vi "Find Car Control VI.vi"(11 "Project":refnum<vi>) -> (0 "error out":errorcluster, 3 "Car Control VI Path":path)   [LabVIEW 2020]
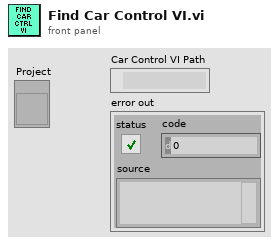
[diagram p1: front panel]
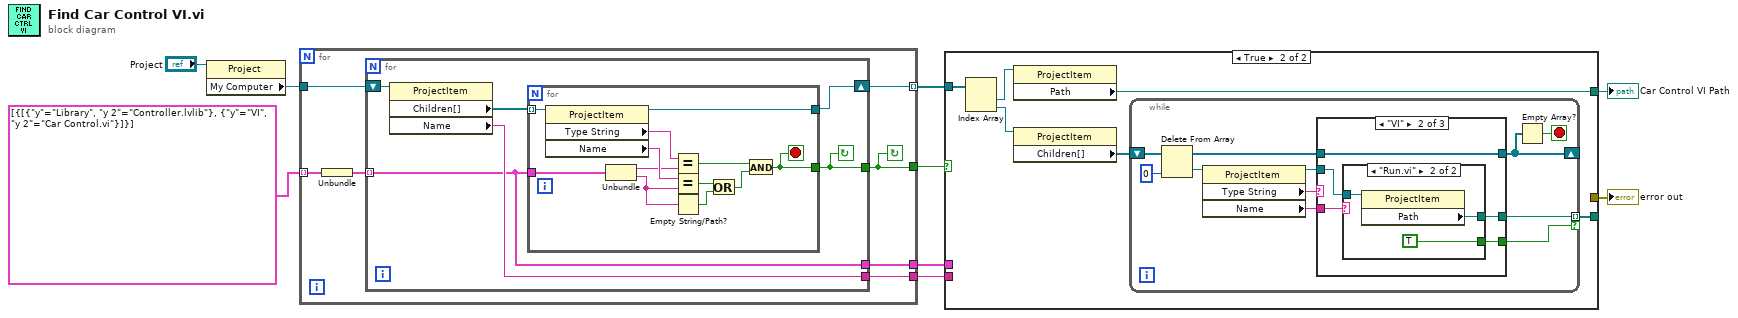
[diagram p0: block diagram]
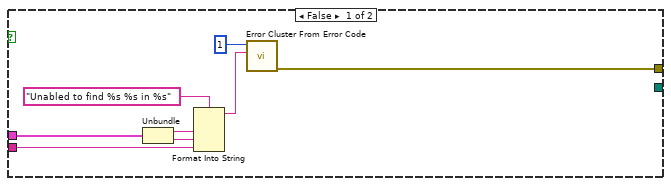
[diagram p2: hidden frame]
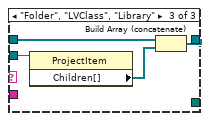
[diagram p5: hidden frame]
diagram:
  n1 = property class="Project"(reference="Project") -> ("My Computer"=w9:refnum<vi>)  [unwired: 1 in, 2 out]
  n2 = for {
    tunnel: w9 -> [w16]
    tunnel: cluster{cluster{"y":string, "y 2":string}[]}[] [{[{"y"="Library", "y 2"="Controller.lvlib"}, {"y"="VI", "y 2"="Car Control.vi"}]}] -> [w15] mode=indexing
    tunnel: [w13] -> w6 mode=indexing
    tunnel: [w12] -> w5
    tunnel: [w11] -> w3
    tunnel: [w10] -> w4
    stop <- w12 continue-if-true
    n3 = Unbundle(w15) -> (w14:cluster{"y":string, "y 2":string}[])
    n4 = for {
      shift-right: [w20] -> w13
      shift-left: w16 -> [w22]
      tunnel: w14 -> [w17] mode=indexing
      tunnel: [w19] -> w12
      tunnel: [w18] -> w11
      tunnel: [w17] -> w10
      stop <- w19 continue-if-true
      n5 = property class="ProjectItem"(reference=w22) -> ("Children[]"=w21:refnum<vi>[], "Name"=w18:string)  [unwired: 1 in, 2 out]
      n6 = for {
        tunnel: w21 -> [w34] mode=indexing
        tunnel: [w32] -> w20
        tunnel: w17 -> [w28]
        tunnel: [w26] -> w19
        stop <- w26 stop-if-true
        n7 = property class="ProjectItem"(reference=w34) -> (reference out=w32:refnum<vi>, "Type String"=w33:string, "Name"=w31:string)  [unwired: 1 in, 1 out]
        n8 = Unbundle(w28) -> ("y"=w27:string, "y 2"=w25:string)
        n9 = Equal?(x=w33, y=w27) -> (x = y?=w30:bool)
        n10 = Equal?(x=w31, y=w25) -> (x = y?=w29:bool)
        n11 = Empty String/Path?(string/path=w25) -> (empty?=w23:bool)
        n12 = Or(x=w29, y=w23) -> (x .or. y?=w24:bool)
        n13 = And(x=w30, y=w24) -> (x .and. y?=w26:bool)
      }
    }
  }
  n14 = case shown="True" w5 {
    tunnel: w6 -> [_ w48]
    tunnel: w4 -> [w40 _]
    tunnel: w3 -> [w37 _]
    tunnel: [w35 _] -> w1
    tunnel: [_ w46] -> w2
    tunnel: [_ w43] -> _
    frame False {
      n15 = Unbundle(w40) -> ("y"=w39:string, "y 2"=w38:string)
      n16 = Format Into String(format string="Unabled to find %s %s in %s", w39, w38, w37) -> (resulting string=w36:string)  [unwired: 2 in, 1 out]
      n17 = call <vilib>:"Error Cluster From Error Code.vi"("error message (\"\")"=w36, "error code (0)"=1) -> ("error out"=w35:errorcluster)  [unwired: 7 in]
    }
    frame True {
      n18 = Index Array(array=w48) -> (element #1=w47:refnum<vi>, element #2=w45:refnum<vi>)  [unwired: 2 in]
      n19 = property class="ProjectItem"(reference=w47) -> ("Path"=w46:path)  [unwired: 1 in, 2 out]
      n20 = property class="ProjectItem"(reference=w45) -> ("Children[]"=w44:refnum<vi>[])  [unwired: 1 in, 2 out]
      n21 = while {
        shift-right: [w53] -> _
        shift-left: w44 -> [w59]
        tunnel: [w50] -> w43 mode=indexing if=w49
        stop <- w52 stop-if-true
        n22 = Delete From Array(array=w59, index=0) -> (deleted portion=w57:refnum<vi>, array with subset deleted=w55:refnum<vi>[])  [unwired: 1 in]
        n23 = property class="ProjectItem"(reference=w57) -> (reference out=w54:refnum<vi>, "Type String"=w56:string, "Name"=w51:string)  [unwired: 1 in, 1 out]
        n24 = case shown="\"VI\"" w56 {
          tunnel: w55 -> [w60 w64 w71]
          tunnel: [w60 w64 w69] -> w53
          tunnel: w54 -> [_ w63 w72]
          tunnel: w51 -> [_ w65 _]
          tunnel: [_ w62 _] -> w50
          tunnel: [_ w61 _] -> w49
          frame Default {
          }
          frame "VI" {
            n25 = case shown="\"Run.vi\"" w65 {
              tunnel: w63 -> [_ w68]
              tunnel: [_ w67] -> w62
              tunnel: [_ TRUE] -> w61
              frame "False", Default {
              }
              frame "Run.vi" {
                n26 = property class="ProjectItem"(reference=w68) -> ("Path"=w67:path)  [unwired: 1 in, 2 out]
              }
            }
          }
          frame "Folder", "LVClass", "Library" {
            n27 = property class="ProjectItem"(reference=w72) -> ("Children[]"=w70:refnum<vi>[])  [unwired: 1 in, 2 out]
            n28 = Build Array (concatenate)(w71, w70) -> (w69:refnum<vi>[])
          }
        }
        n29 = Empty Array?(array=w53) -> (empty?=w52:bool)
      }
    }
  }
  "Car Control VI Path" <- w2
  "error out" <- w1
